vi "target - single rate - variables.vi"() -> ()   [LabVIEW 2017]
uses:
  <vilib>/Platform/TimedLoop/XDataNode/timing_clust.ctl
  <vilib>/Platform/TimedLoop/XDataNode/nitl_modes.ctl
  <vilib>/Platform/TimedLoop/XDataNode/wakeup.ctl
  <vilib>/Platform/TimedLoop/XDataNode/XDataNode.xnode
  <vilib>/Platform/TimedLoop/XDataNode/XDNodeRunTimeDep.lvlib
panel:
  out "value":dbl
  in  "stop":bool
  out "Time lapsed":u32
  out "Loop counter":i32
  in  "Upload to pc cycle":i32
  in  "On/~Off":bool
  in  "Enable/~Disable":bool
  in  "Forward/~Backward":bool
  out "State":bool[](array[boolean])
  # "The Network Variable Engine and Variable Client Support must be installed on the RT target\nfor this application to function properly. If the Network Variable Engine is not supported on\nthe target (e.g.  FP-2000 with <32MB of RAM), open the project and move the variable library\nto My Computer in the project. Doing this will deploy the variables to localhost but\nwill still require that Variable Client Support be installed on the RT target."
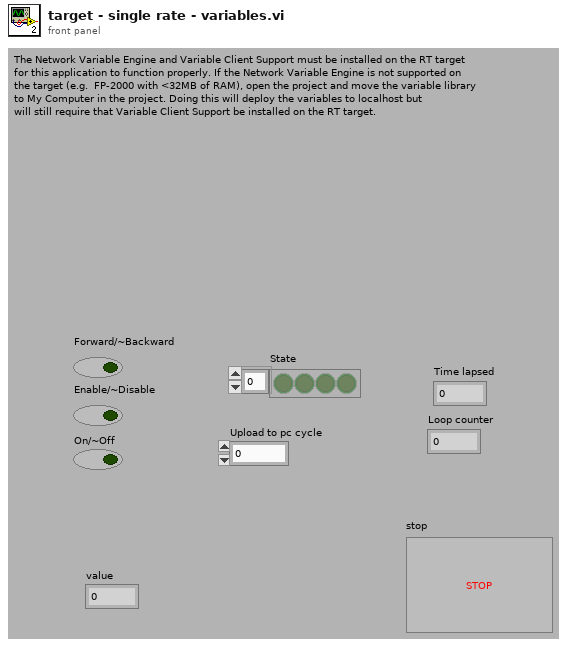
[diagram p1: front panel]
types:
  T1 = typedef "XDNodeRunTimeDep.lvlib/timing_clust.ctl" = cluster{"Expected End [f-1]":u64, "Actual End [f-1]":u64, "Finished Late? [f-1]":bool, "Expected End [i-1]":u64, "Actual End [i-1]":u64, "Finished Late? [i-1]":bool, "Expected Start [i]":u64, "Actual Start [i]":u64, "Expected Start [f]":u64, "Actual Start [f]":u64, "Source Name":string, "Structure Name":string, "Period":i64, "Deadline":i64, "Offset":i64, "Start":i64, "Priority":i32, "Timeout":i32, "Mode":T2, "Wakeup Reason":T3, "Error":errorcluster, "Source Type":string, "Secondary Source Type":string, "Global End Time":u64, "Global Start Time":u64, "Frame Duration":u64, "Iteration Duration":u64, "Assigned CPU":i32, "I/O Scan Engine Mode":u32}
  T2 = typedef "XDNodeRunTimeDep.lvlib/nitl_modes.ctl" = enum32{"No Change", "Process missed periods, maintain original phase", "Discard missed periods, maintain original phase", "Process missed periods, ignore original phase", "Discard missed periods, ignore original phase"}
  T3 = typedef "XDNodeRunTimeDep.lvlib/wakeup.ctl" = enum32{"Normal", "Aborted", "Asynchronous wakeup", "Timing source error", "Timed loop error", "Timeout"}
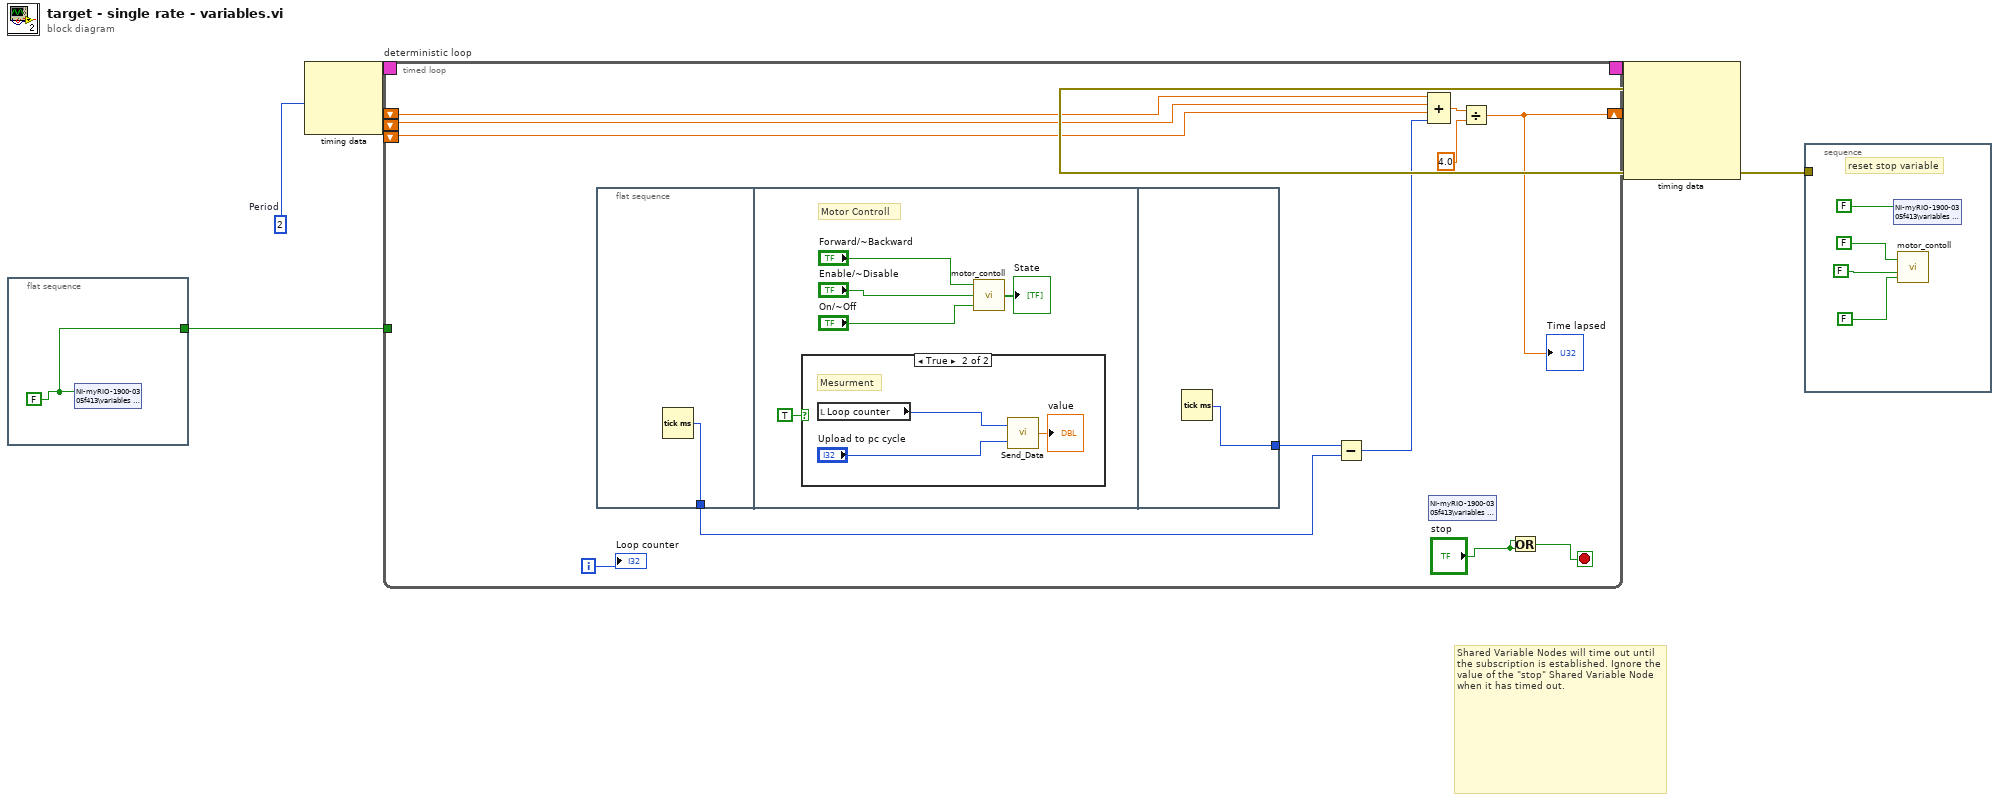
[diagram p0: block diagram]
diagram:
  w3 = i64 2  # Period
  # "Shared Variable Nodes will time out until the subscription is established. Ignore the value of the \"stop\" Shared Variable Node when it has timed out."
  n1 = flat-sequence {
    tunnel: [w6] -> w1
    frame #0 {
      w6 = FALSE
      n2 = shared-variable "NI-myRIO-1900-0305f413\\variables - network - RT.lvlib\\stop"(w6) -> ()  [unwired: 1 in, 1 out]
    }
  }
  n3 = node-c288 ("Input Node")(w3) -> (w5:T1)  [unwired: 2 in]
  n4 = timed-loop "deterministic loop" {
    timing: w5 -> [_]
    timing-out: [_] -> w4
    shift-right: [w9] -> _
    shift-left: _ -> [w15]
    shift-left: _ -> [w11]
    shift-left: _ -> [w10]
    tunnel: w1 -> [_]
    i -> [w18]
    stop <- w8 stop-if-true
    n5 = flat-sequence {
      tunnel: [w19] -> w16
      tunnel: [w28] -> w17
      frame #0 {
        n6 = Tick Count (ms)() -> (millisecond timer value=w19:u32)
      }
      frame #1 {
        # "Motor Controll"
        n7 = case shown="True" TRUE {
          frame False {
          }
          frame True {
            # "Mesurment"
            n8 = local read "Loop counter"() -> (w26:i32)
            n9 = call "Send_Data.vi"("Upload to pc cycle"="Upload to pc cycle", "Counter"=w26) -> ("value"=→"value":dbl)
          }
        }
        n10 = call "motor_contoll.vi"("On/Off"="On/~Off", "Enable/Disable"="Enable/~Disable", "Forward/Backward"="Forward/~Backward") -> ("State"=→"State":bool[])
      }
      frame #2 {
        n11 = Tick Count (ms)() -> (millisecond timer value=w28:u32)
      }
    }
    n12 = Subtract(x=w17, y=w16) -> (x-y=w13:u32)
    n13 = Compound Arithmetic op=ADD(w15, w11, w10, w13) -> (w14:dbl)
    n14 = shared-variable "NI-myRIO-1900-0305f413\\variables - network - RT.lvlib\\stop"() -> ()  [unwired: 1 in, 2 out]
    n15 = Divide(x=w14, y=4.0) -> (x/y=w9:dbl)
    "Time lapsed" <- w9
    n16 = Or(x="stop", y="stop") -> (x .or. y?=w8:bool)
    "Loop counter" <- w18
  }
  n17 = node-c288 ("Output Node")(w4) -> (w2:errorcluster)  [unwired: 5 out]
  n18 = stacked-sequence {
    tunnel: w2 -> [_]
    frame #0 {
      # "reset stop variable"
      n19 = shared-variable "NI-myRIO-1900-0305f413\\variables - network - RT.lvlib\\stop"(FALSE) -> ()  [unwired: 1 in, 1 out]
      n20 = call "motor_contoll.vi"("On/Off"=FALSE ("On/~Off"), "Enable/Disable"=FALSE ("Enable/~Disable"), "Forward/Backward"=FALSE ("Forward/~Backward")) -> ()  [unwired: 1 out]
    }
  }
